vi "ConstructorString.vi"(6 "error in":errorcluster, 9 "Structure in":refnum<class "Structure.lvclass">) -> (0 "error out":errorcluster, 3 "Structure out":refnum<class "Structure.lvclass">, 4 "constructor":string)   [LabVIEW 2014, in "Structure.lvclass"]
uses:
  Structure.lvclass
  Python/Parsing/ListTypesTD.ctl
  Python/Parsing/Python Functions.lvlib
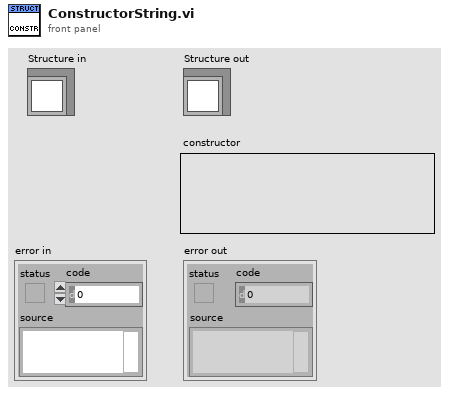
[diagram p1: front panel]
types:
  T1 = typedef "Python Functions.lvlib/ListTypesTD.ctl" = enum16{"list", "tuple", "parameter list", "output list"}
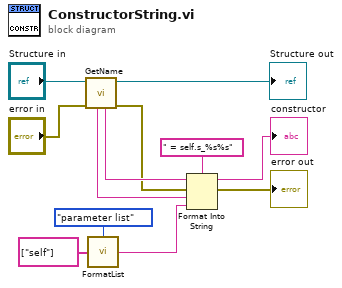
[diagram p0: block diagram]
diagram:
  n1 = call-dynamic "GetName.vi"("error in"="error in", "Structure in"="Structure in") -> ("error out"=w1:errorcluster, "Structure out"=→"Structure out":refnum<class "Structure.lvclass">, "name"=w4:string, "UID"=w3:string)  [unwired: 4 in]
  n2 = call "FormatList.vi"("values"=string[] ["self"], "type"=ListTypesTD."parameter list") -> ("python object"=w10:string)
  n3 = Format Into String(format string=" = self.s_%s%s", initial string=w4, error in=w1, w3, w10) -> (resulting string=→"constructor":string, error out=→"error out":errorcluster)
